vi "load_config_thesvi.vi"(8 "Config Directory":path=path "D:/ParDates") -> (10 "Noff":u32 step=1, 12 "USED_FILTERS":u8[](array[numeric]), 14 "USED_LEDS":bool[][](array[boolean]), 15 "NPAT":u32, 16 "EXPT":dbl, 17 "BETWEEN_SCAN":u32, 18 "Non":u32=150 step=1, 19 "NSCAN":u32, 20 "Refnum VISA en sortie":refnum<visa-resource-name>="COM1", 21 "BIN":u16, 22 "Nstart":u32=30 step=1, 23 "ROMODE":u32, 24 "BETWEEN_PAT":u32, 25 "STAGE_SPEED":dbl, 26 "XYPOS":T1)   [LabVIEW 2013]
uses:
  <vilib>/Analysis/Matrix/Datatypes/RealMatrix.ctl
  <vilib>/Analysis/Matrix/NI_Matrix.lvlib
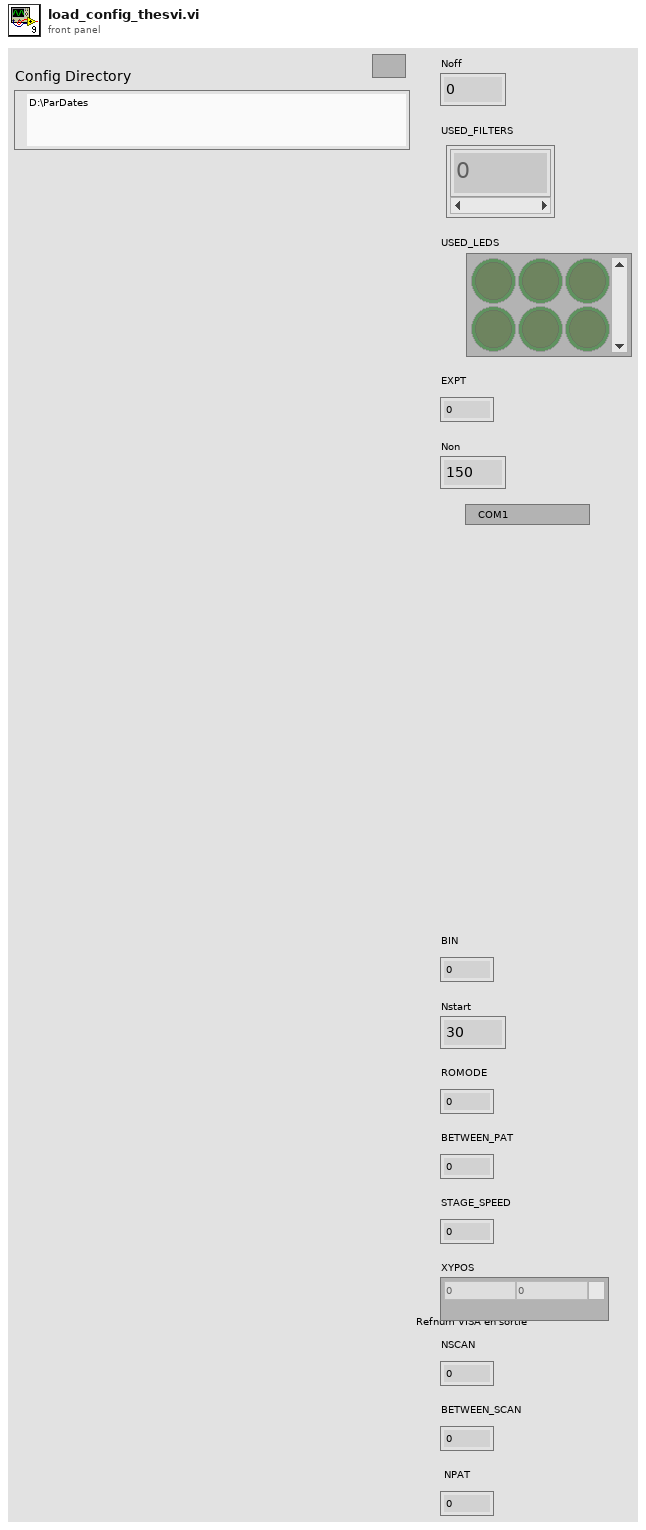
[diagram p1: front panel]
types:
  T1 = typedef "NI_Matrix.lvlib/RealMatrix.ctl" = dbl[][]
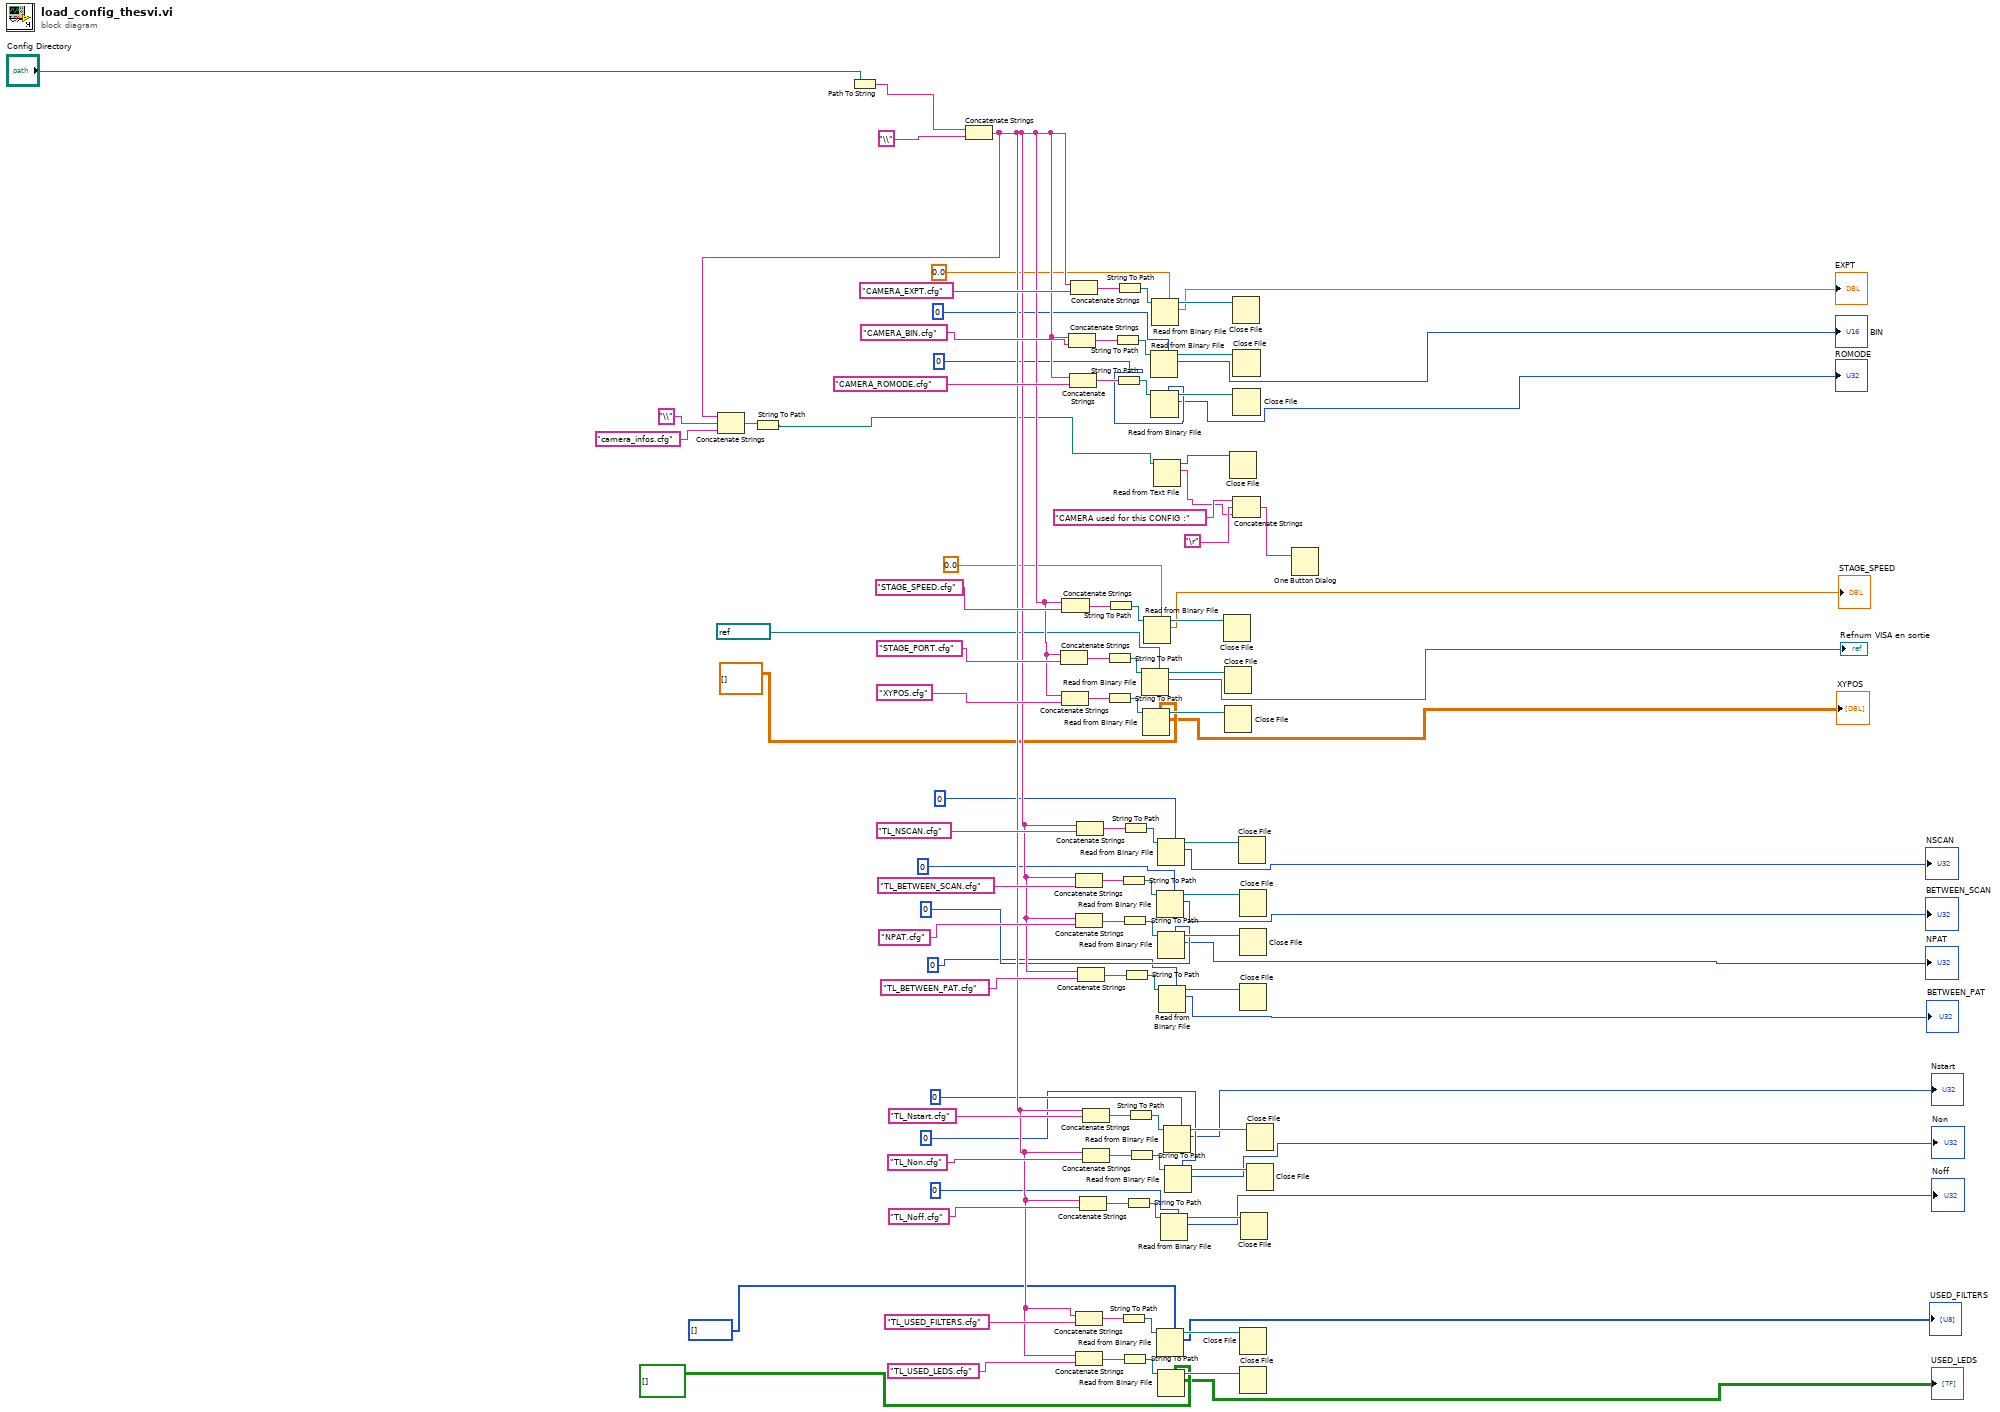
[diagram p0: block diagram]
diagram:
  n1 = Path To String(path="Config Directory") -> (string=w37:string)
  n2 = Concatenate Strings(w37, "\\") -> (w41:string)
  n3 = Concatenate Strings(w41, "\\", "camera_infos.cfg") -> (w40:string)
  n4 = String To Path(string=w40) -> (path=w36:path)
  n5 = Concatenate Strings(w41, "STAGE_PORT.cfg") -> (w88:string)
  n6 = Concatenate Strings(w41, "XYPOS.cfg") -> (w87:string)
  n7 = Concatenate Strings(w41, "STAGE_SPEED.cfg") -> (w89:string)
  n8 = Concatenate Strings(w41, "CAMERA_BIN.cfg") -> (w98:string)
  n9 = Concatenate Strings(w41, "CAMERA_ROMODE.cfg") -> (w94:string)
  n10 = Concatenate Strings(w41, "CAMERA_EXPT.cfg") -> (w99:string)
  n11 = Concatenate Strings(w41, "TL_BETWEEN_SCAN.cfg") -> (w76:string)
  n12 = Concatenate Strings(w41, "TL_USED_FILTERS.cfg") -> (w58:string)
  n13 = Concatenate Strings(w41, "NPAT.cfg") -> (w75:string)
  n14 = Concatenate Strings(w41, "TL_USED_LEDS.cfg") -> (w57:string)
  n15 = Concatenate Strings(w41, "TL_NSCAN.cfg") -> (w77:string)
  n16 = Concatenate Strings(w41, "TL_BETWEEN_PAT.cfg") -> (w68:string)
  n17 = Concatenate Strings(w41, "TL_Noff.cfg") -> (w59:string)
  n18 = Concatenate Strings(w41, "TL_Nstart.cfg") -> (w67:string)
  n19 = Concatenate Strings(w41, "TL_Non.cfg") -> (w66:string)
  n20 = String To Path(string=w88) -> (path=w85:path)
  n21 = String To Path(string=w87) -> (path=w84:path)
  n22 = String To Path(string=w89) -> (path=w86:path)
  n23 = String To Path(string=w98) -> (path=w97:path)
  n24 = String To Path(string=w94) -> (path=w93:path)
  n25 = String To Path(string=w99) -> (path=w101:path)
  n26 = String To Path(string=w76) -> (path=w73:path)
  n27 = String To Path(string=w58) -> (path=w55:path)
  n28 = String To Path(string=w75) -> (path=w72:path)
  n29 = String To Path(string=w57) -> (path=w54:path)
  n30 = String To Path(string=w77) -> (path=w74:path)
  n31 = String To Path(string=w68) -> (path=w65:path)
  n32 = String To Path(string=w59) -> (path=w56:path)
  n33 = String To Path(string=w67) -> (path=w64:path)
  n34 = String To Path(string=w66) -> (path=w63:path)
  n35 = Read from Binary File(5:refnum<visa-resource-name> "COM1" ("STAGE_PORT 2"), 11:w85) -> (2:→"Refnum VISA en sortie":refnum<visa-resource-name>, 3:w82:refnum<file>)  [unwired: 4 in, 2 out]
  n36 = Read from Binary File(5:T1 [] ("XYPOS 2"), 11:w84) -> (2:→"XYPOS":T1, 3:w81:refnum<file>)  [unwired: 4 in, 2 out]
  n37 = Read from Binary File(5:0.0, 11:w86) -> (2:→"STAGE_SPEED":dbl, 3:w83:refnum<file>)  [unwired: 4 in, 2 out]
  n38 = Read from Binary File(5:u16 0, 11:w97) -> (2:→"BIN":u16, 3:w91:refnum<file>)  [unwired: 4 in, 2 out]
  n39 = Read from Binary File(5:u32 0, 11:w93) -> (2:→"ROMODE":u32, 3:w90:refnum<file>)  [unwired: 4 in, 2 out]
  n40 = Read from Binary File(5:0.0, 11:w101) -> (2:→"EXPT":dbl, 3:w92:refnum<file>)  [unwired: 4 in, 2 out]
  n41 = Read from Text File(file (use dialog)=w36) -> (refnum out=w35:refnum<file>, text=w32:string)  [unwired: 3 in, 2 out]
  n42 = Read from Binary File(5:u32 0, 11:w73) -> (2:→"BETWEEN_SCAN":u32, 3:w70:refnum<file>)  [unwired: 4 in, 2 out]
  n43 = Read from Binary File(5:u8[] [] ("USED_FILTERS 2"), 11:w55) -> (2:→"USED_FILTERS":u8[], 3:w52:refnum<file>)  [unwired: 4 in, 2 out]
  n44 = Read from Binary File(5:u32 0, 11:w72) -> (2:→"NPAT":u32, 3:w69:refnum<file>)  [unwired: 4 in, 2 out]
  n45 = Read from Binary File(5:bool[][] [] ("USED_LEDS 2"), 11:w54) -> (2:→"USED_LEDS":bool[][], 3:w51:refnum<file>)  [unwired: 4 in, 2 out]
  n46 = Read from Binary File(5:u32 0, 11:w74) -> (2:→"NSCAN":u32, 3:w71:refnum<file>)  [unwired: 4 in, 2 out]
  n47 = Read from Binary File(5:u32 0, 11:w65) -> (2:→"BETWEEN_PAT":u32, 3:w62:refnum<file>)  [unwired: 4 in, 2 out]
  n48 = Read from Binary File(5:u32 0, 11:w56) -> (2:→"Noff":u32, 3:w53:refnum<file>)  [unwired: 4 in, 2 out]
  n49 = Read from Binary File(5:u32 0, 11:w64) -> (2:→"Nstart":u32, 3:w61:refnum<file>)  [unwired: 4 in, 2 out]
  n50 = Read from Binary File(5:u32 0, 11:w63) -> (2:→"Non":u32, 3:w60:refnum<file>)  [unwired: 4 in, 2 out]
  n51 = Close File(refnum=w83) -> ()  [unwired: 1 in, 2 out]
  n52 = Close File(refnum=w82) -> ()  [unwired: 1 in, 2 out]
  n53 = Close File(refnum=w81) -> ()  [unwired: 1 in, 2 out]
  n54 = Close File(refnum=w35) -> ()  [unwired: 1 in, 2 out]
  n55 = Close File(refnum=w92) -> ()  [unwired: 1 in, 2 out]
  n56 = Close File(refnum=w91) -> ()  [unwired: 1 in, 2 out]
  n57 = Close File(refnum=w90) -> ()  [unwired: 1 in, 2 out]
  n58 = Concatenate Strings("CAMERA used for this CONFIG :", "\r", w32) -> (w31:string)
  n59 = Close File(refnum=w71) -> ()  [unwired: 1 in, 2 out]
  n60 = Close File(refnum=w70) -> ()  [unwired: 1 in, 2 out]
  n61 = Close File(refnum=w69) -> ()  [unwired: 1 in, 2 out]
  n62 = Close File(refnum=w62) -> ()  [unwired: 1 in, 2 out]
  n63 = Close File(refnum=w52) -> ()  [unwired: 1 in, 2 out]
  n64 = Close File(refnum=w51) -> ()  [unwired: 1 in, 2 out]
  n65 = Close File(refnum=w53) -> ()  [unwired: 1 in, 2 out]
  n66 = Close File(refnum=w61) -> ()  [unwired: 1 in, 2 out]
  n67 = Close File(refnum=w60) -> ()  [unwired: 1 in, 2 out]
  n68 = One Button Dialog(message=w31) -> ()  [unwired: 1 in, 1 out]
